vi "FitLorentzian.vi"() -> ()   [LabVIEW 2014]
uses:
  <vilib>/Utility/file.llb/Read Delimited Spreadsheet (DBL).vi
  <vilib>/gmath/NI_Gmath.lvlib
  <vilib>/gmath/NumericalOptimization/Nonlinear Curve Fit LM.vi
  <vilib>/Analysis/NI_AALBase.lvlib
  <vilib>/Analysis/baseanly.llb/Mean (DBL).vi
panel:
  out "Parameter Guess":dbl[](array[numeric]) caption="pos\nwidth\namplitude*\noffset" format="%.4e"
  out "best fit parameters":dbl[](array[numeric]) caption="pos\nwidth\nheight\noffset" format="%.4e"
  out "XY Graph":cluster{cdb[]}[](graph)
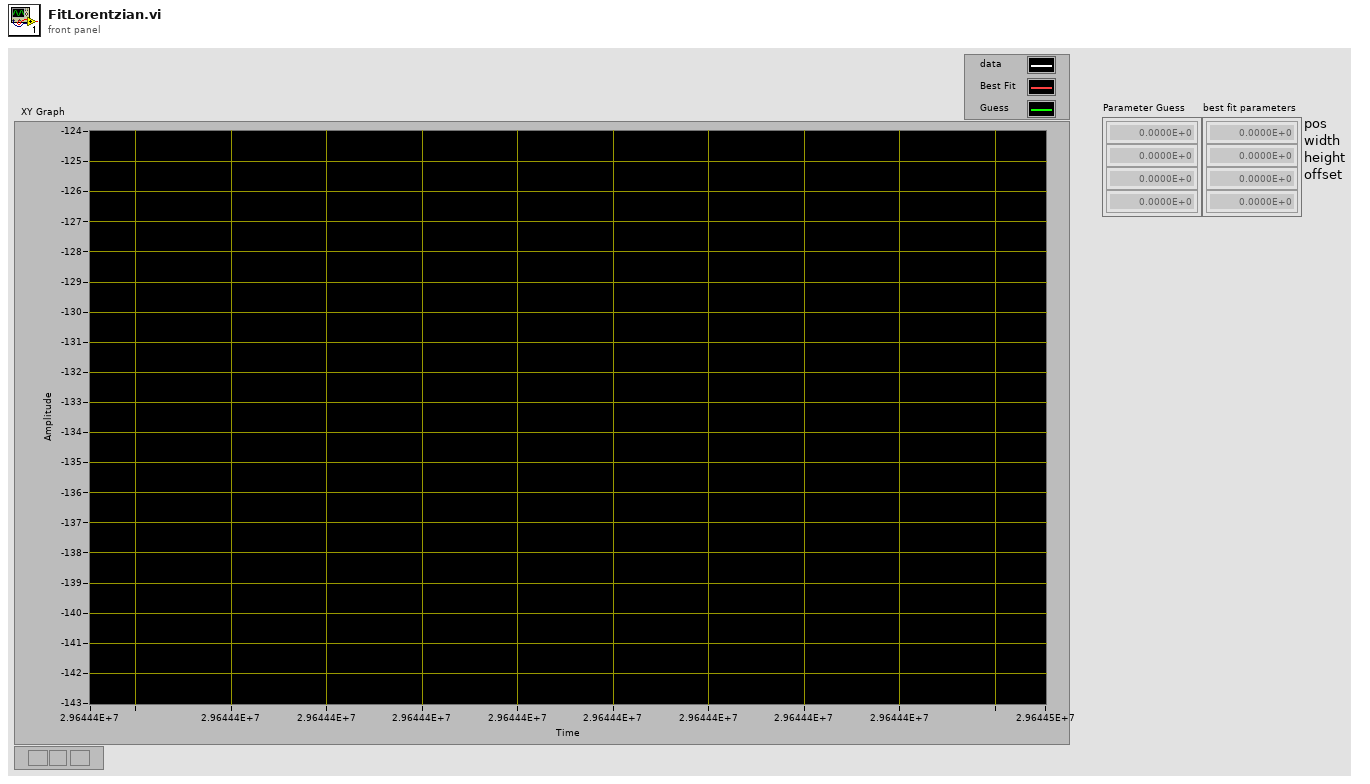
[diagram p1: front panel]
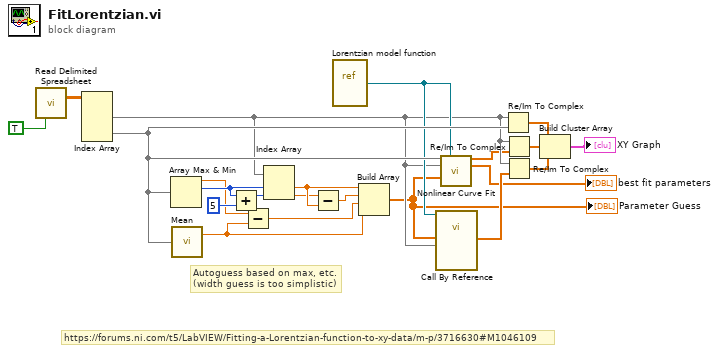
[diagram p0: block diagram]
diagram:
  # "https://forums.ni.com/t5/LabVIEW/Fitting-a-Lorentzian-function-to-xy-data/m-p/3716630#M1046109"
  # "Autoguess based on max, etc.\n(width guess is too simplistic)"
  n1 = call-poly <vilib>:"Read Delimited Spreadsheet.vi"("transpose? (F)"=TRUE) -> ("all rows"=w21:dbl[][])  [unwired: 9 in, 5 out]
  n2 = Index Array(array=w21) -> (element #1=w10:dbl[], element #2=w19:dbl[])  [unwired: 4 in]
  n3 = Array Max & Min(array=w19) -> (max value=w3:dbl, max index (indices)=w18:i32)  [unwired: 2 out]
  n4 = call-poly <vilib>:"Mean.vi"("X"=w19) -> ("mean"=w4:dbl)  [unwired: 1 out]
  n5 = Add(x=w18, y=5) -> (x+y=w17:i32)
  n6 = Subtract(x=w3, y=w4) -> (x-y=w1:dbl)
  n7 = Index Array(array=w10, index #1=w18, index #2=w17) -> (element #1=w15:dbl, element #2=w14:dbl)
  n8 = Subtract(x=w14, y=w15) -> (x-y=w12:dbl)
  n9 = vi-ref "Lorentzian model function.vi"() -> (w11:refnum<vi>)
  n10 = Build Array(w15, w12, w1, w4) -> (w2:dbl[])
  "Parameter Guess" <- w2
  n11 = call-by-ref "?"(reference=w11, "X"=w10, "a"=w2) -> ("f(X,a)"=w8:dbl[])  [unwired: 3 in, 4 out]
  n12 = call-poly <vilib>:"Nonlinear Curve Fit.vi"("Y"=w19, "f(x,a)"=w11, "X"=w10, "initial parameters"=w2) -> ("best nonlinear fit"=w6:dbl[], "best fit parameters"=→"best fit parameters":dbl[])  [unwired: 6 in, 4 out]
  n13 = Re/Im To Complex(1:w19, 2:w10) -> (0:w20:cdb[])
  n14 = Re/Im To Complex(1:w6, 2:w10) -> (0:w9:cdb[])
  n15 = Re/Im To Complex(1:w8, 2:w10) -> (0:w7:cdb[])
  n16 = Build Cluster Array(w20, w9, w7) -> (→"XY Graph":cluster{cdb[]}[])
